vi "SignalToNode(viaString).vi"(0 "Tree DVR in":refnum<data-value>, 1 "NodePath":string, 2 "y-axis (Data Range)":dbl[](array[numeric]), 3 "Start Time":dbl, 4 "Delta t":dbl, 5 "error in (no error)":errorcluster) -> (6 "Tree DVR out":refnum<data-value>, 8 "error out":errorcluster)   [LabVIEW 2011]
uses:
  <vilib>/MDSplus/Classes/Tree_Class/Tree.lvclass
  <vilib>/MDSplus/Library/MDSplus.lvlib
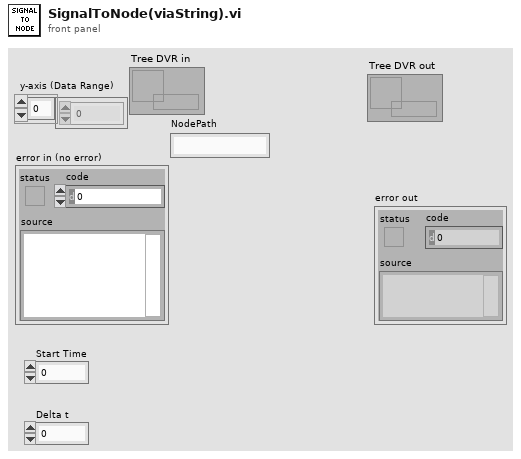
[diagram p1: front panel]
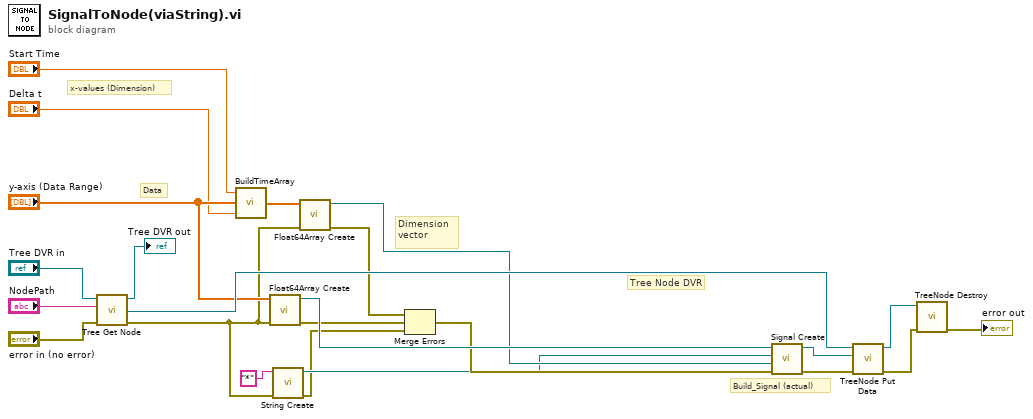
[diagram p0: block diagram]
diagram:
  # "Build_Signal (actual)"
  # "Dimension vector"
  # "x-values (Dimension)"
  # "Tree Node DVR"
  # "Data"
  n1 = call <vilib>:"Tree Get Node.vi"("error in (no error)"="error in (no error)", "Path"="NodePath", "Tree DVR in"="Tree DVR in") -> ("error out"=w5:errorcluster, "Node out"=w20:refnum<data-value>, "Tree DVR out"=→"Tree DVR out":refnum<data-value>)  [unwired: 6 in]
  n2 = call "BuildTimeArray.vi"("Time Increment (dt)"="Delta t", "Data Array (y-values)"="y-axis (Data Range)", "Start Time (t_o)"="Start Time") -> ("Time Array (x-values)"=w11:dbl[])
  n3 = call <vilib>:"Float64Array Create.vi"("error in (no error)"=w5, "DBL array in"="y-axis (Data Range)") -> ("error out"=w17:errorcluster, "Float64Array DVR out"=w18:refnum<data-value>)  [unwired: 8 in]
  n4 = call <vilib>:"String Create.vi"("error in (no error)"=w5, "String value in"="*") -> ("error out"=w6:errorcluster, "String DVR out"=w7:refnum<data-value>)  [unwired: 8 in]
  n5 = call <vilib>:"Float64Array Create.vi"("error in (no error)"=w5, "DBL array in"=w11) -> ("error out"=w10:errorcluster, "Float64Array DVR out"=w9:refnum<data-value>)  [unwired: 8 in]
  n6 = Merge Errors(w10, w17, w6) -> (w15:errorcluster)
  n7 = call <vilib>:"Signal Create.vi"("error in (no error)"=w15, "Dimension"=w9, "Raw"=w7, "Data"=w18) -> ("error out"=w19:errorcluster, "Signal DVR out"=w16:refnum<data-value>)  [unwired: 6 in]
  n8 = call <vilib>:"TreeNode Put Data.vi"("error in (no error)"=w19, "Data"=w16, "TreeNode DVR in"=w20) -> ("error out"=w3:errorcluster, "TreeNode DVR out"=w4:refnum<data-value>)  [unwired: 7 in]
  n9 = call <vilib>:"TreeNode Destroy.vi"("error in (no error)"=w3, "TreeNode DVR in"=w4) -> ("error out"=→"error out":errorcluster)  [unwired: 9 in]
